vi "DatawarehouseProperty.vi"   [LabVIEW 2021]
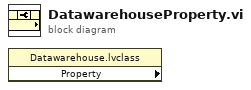
[diagram p0: block diagram]
diagram:
  n1 = property class="Datawarehouse.lvclass" props=[]() -> ()  [unwired: 2 in, 3 out]
